vi "Validate_VI_Can_Be_Inlined_In_Build.vi"(5 "topLevel":bool, 6 "VI refnum in":refnum<vi>, 7 "sourceInclusion":T1, 8 "error in (no error)":errorcluster, 10 "saveLevel":u32, 11 "Build in":refnum<class "AB_SourceDistribution.lvclass">) -> (0 "error out":errorcluster, 3 "Build out":refnum<class "AB_SourceDistribution.lvclass">)   [LabVIEW 2020, in "AB_SourceDistribution.lvclass"]
uses:
  <vilib>/AppBuilder/AB_Classes/SourceDistribution/AB_SourceDistribution.lvclass
  <vilib>/AppBuilder/AB_Source_Inclusion.ctl
  <resource>/Framework/Providers/Common/provcom_StringGlobals.vi
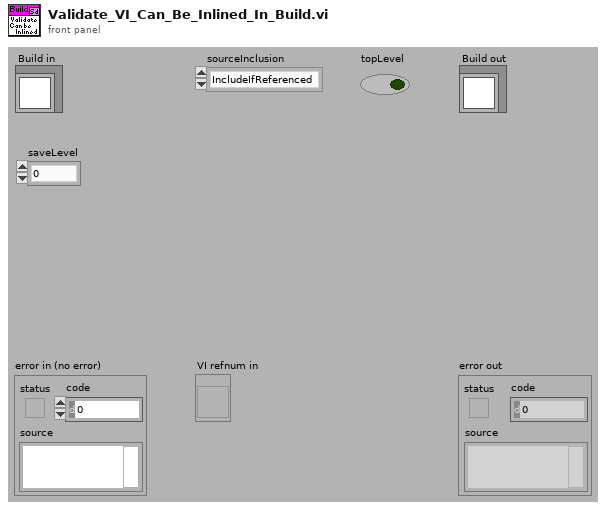
[diagram p1: front panel]
types:
  T1 = typedef "AB_Source_Inclusion.ctl" = enum16{"IncludeIfReferenced", "Include", "Exclude", "TopLevel"}
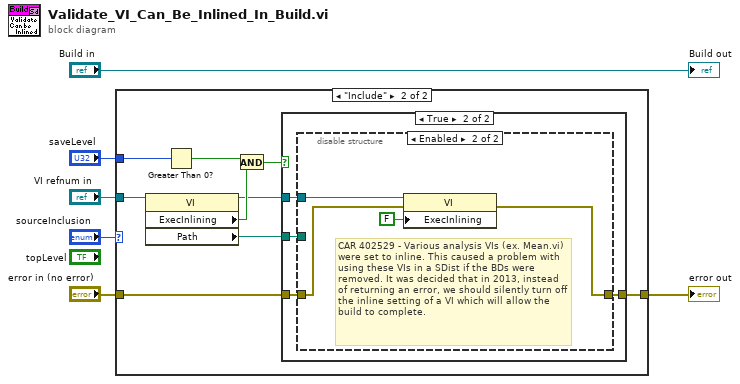
[diagram p0: block diagram]
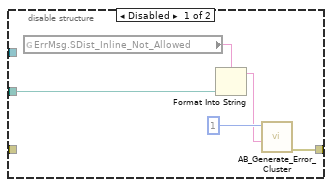
[diagram p4: hidden frame]
diagram:
  n1 = case shown="\"Include\"" "sourceInclusion" {
    tunnel: "saveLevel" -> [_ w16]
    tunnel: "error in (no error)" -> [w7 w13]
    tunnel: [w7 w12] -> w3
    tunnel: "VI refnum in" -> [_ w11]
    frame Default {
    }
    frame "Include" {
      n2 = property class="VI"(reference=w11) -> (reference out=w8:refnum<vi>, "ExecInlining"=w9:bool, "Path"=w10:path)  [unwired: 1 in, 1 out]
      n3 = Greater Than 0?(x=w16) -> (x > 0?=w15:bool)
      n4 = And(x=w15, y=w9) -> (x .and. y?=w14:bool)
      n5 = case shown="True" w14 {
        tunnel: w13 -> [w17 w18]
        tunnel: [w17 w21] -> w12
        tunnel: w10 -> [_ w20]
        tunnel: w8 -> [_ w19]
        frame False {
        }
        frame True {
          n6 = disable-structure shown="Enabled" {
            disable-tunnel: [w26 w27] -> w21
            disable-tunnel: w20 -> [w22 _]
            disable-tunnel: w19 -> [_ w29]
            disable-tunnel: w18 -> [_ w28]
            frame Disabled {
              n7 = global read "provcom_StringGlobals.vi" "ErrMsg.SDist_Inline_Not_Allowed"() -> (w24:string)
              n8 = Format Into String(format string=w24, w22) -> (resulting string=w23:string)  [unwired: 2 in, 1 out]
              n9 = call <vilib>:"AB_Generate_Error_Cluster.vi"("Additional Message"=w23, "Code"=1) -> ("error out"=w26:errorcluster)  [unwired: 2 in, 7 out]
            }
            frame Enabled {
              # "CAR 402529 - Various analysis VIs (ex. Mean.vi) were set to inline. This caused a problem with using these VIs in a SDist if the BDs were removed. It was decided that in 2013, instead of returning an error, we should silently turn off the inline setting of a VI which will allow the build to complete."
              n10 = property class="VI"(reference=w29, error in=w28, "ExecInlining"=FALSE ("Execution:Inline SubVI")) -> (error out=w27:errorcluster)  [unwired: 1 out]
            }
          }
        }
      }
    }
  }
  "error out" <- w3
  "Build out" <- "Build in"
